vi "Register gRPC Methods.vi"(8 "error in (no error)":errorcluster, 11 "gRPC service in":refnum<class "NI_XNET_CAN_Bus_Monitor_API.lvclass">) -> (0 "error out":errorcluster, 3 "gRPC service out":refnum<class "NI_XNET_CAN_Bus_Monitor_API.lvclass">)   [LabVIEW 2025, in "xnet_can_bus_monitor_api_server.lvlib" / "NI_XNET_CAN_Bus_Monitor_API.lvclass"]
uses:
  NI_XNET_CAN_Bus_Monitor_API.lvclass
  typeDefs/Server Internal UEs.ctl
  typeDefs/Server Internal Message.ctl
  typeDefs/Server gRPC UEs.ctl
  <vilib>/gRPC/LabVIEW gRPC Library/Server API/typeDefs/gRPCId Cluster.ctl
  <vilib>/gRPC/LabVIEW gRPC Library/Shared/grpcId.ctl
  NI_XNET_CAN_Bus_Monitor_API.lvclass/NI_XNET_CAN_Bus_Monitor_API.ctl
  <vilib>/gRPC/LabVIEW gRPC Library/grpc-lvsupport-release.lvlib
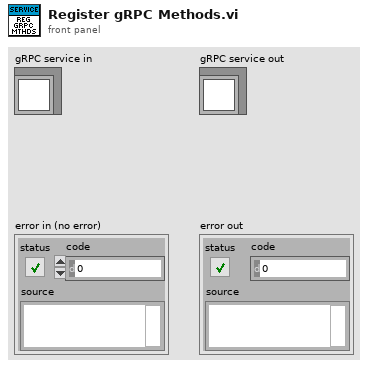
[diagram p1: front panel]
types:
  T1 = typedef "xnet_can_bus_monitor_api_server.lvlib/NI_XNET_CAN_Bus_Monitor_API.lvclass/Server gRPC UEs.ctl" = cluster{"NI_XNET_CAN_Bus_Monitor_API PassThru gRPC UE":refnum<user-event>, "NI_XNET_CAN_Bus_Monitor_API GetStreamingFilter gRPC UE":refnum<user-event>, "NI_XNET_CAN_Bus_Monitor_API SetStreamingFilter gRPC UE":refnum<user-event>, "NI_XNET_CAN_Bus_Monitor_API ResetStreamingFilter gRPC UE":refnum<user-event>, "NI_XNET_CAN_Bus_Monitor_API InitializeSettings gRPC UE":refnum<user-event>, "NI_XNET_CAN_Bus_Monitor_API StopProcess gRPC UE":refnum<user-event>, "NI_XNET_CAN_Bus_Monitor_API StreamBus gRPC UE":refnum<user-event>}
  T2 = typedef "xnet_can_bus_monitor_api_server.lvlib/NI_XNET_CAN_Bus_Monitor_API.lvclass/Server Internal UEs.ctl" = cluster{"NI_XNET_CAN_Bus_Monitor_API PassThru Internal UE":refnum<user-event>, "NI_XNET_CAN_Bus_Monitor_API GetStreamingFilter Internal UE":refnum<user-event>, "NI_XNET_CAN_Bus_Monitor_API SetStreamingFilter Internal UE":refnum<user-event>, "NI_XNET_CAN_Bus_Monitor_API ResetStreamingFilter Internal UE":refnum<user-event>, "NI_XNET_CAN_Bus_Monitor_API InitializeSettings Internal UE":refnum<user-event>, "NI_XNET_CAN_Bus_Monitor_API StopProcess Internal UE":refnum<user-event>, "NI_XNET_CAN_Bus_Monitor_API StreamBus Internal UE":refnum<user-event>}
  T3 = typedef "grpc-lvsupport-release.lvlib/grpcId.ctl" = u64
  T4 = typedef "xnet_can_bus_monitor_api_server.lvlib/NI_XNET_CAN_Bus_Monitor_API.lvclass/Server Internal Message UE.ctl" = refnum<user-event>
  T5 = typedef "grpc-lvsupport-release.lvlib/gRPCId Cluster UE.ctl" = refnum<user-event>
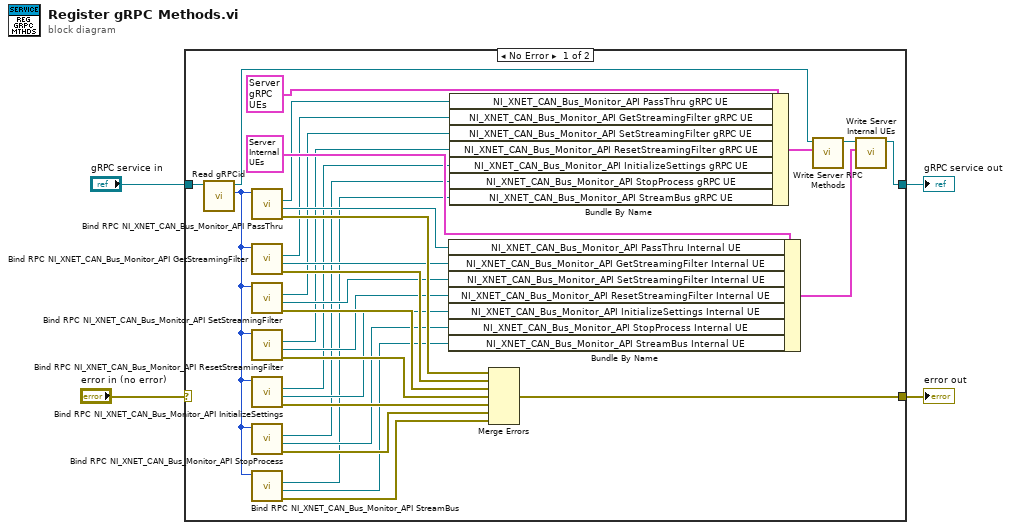
[diagram p0: block diagram]
diagram:
  n1 = case shown="No Error" "error in (no error)" {
    selector: "error in (no error)" -> [_ w36]
    tunnel: "gRPC service in" -> [w27 w37]
    tunnel: [w35 w36] -> w3
    tunnel: [w34 w37] -> w2
    frame No Error {
      n2 = call-dynamic "Read gRPCid.vi"("gRPC service in"=w27) -> ("gRPCid"=w26:T3, "gRPC service out"=w28:refnum<class "NI_XNET_CAN_Bus_Monitor_API.lvclass">)  [unwired: 8 in, 1 out]
      n3 = call "Bind RPC NI_XNET_CAN_Bus_Monitor_API PassThru.vi"("gRPCid server in"=w26) -> ("error out"=w25:errorcluster, "NI_XNET_CAN_Bus_Monitor_API PassThru Internal UE"=w23:T4, "NI_XNET_CAN_Bus_Monitor_API PassThru gRPC UE"=w24:T5)  [unwired: 7 in, 1 out]
      n4 = call "Bind RPC NI_XNET_CAN_Bus_Monitor_API GetStreamingFilter.vi"("gRPCid server in"=w26) -> ("error out"=w22:errorcluster, "NI_XNET_CAN_Bus_Monitor_API GetStreamingFilter Internal UE"=w20:T4, "NI_XNET_CAN_Bus_Monitor_API GetStreamingFilter gRPC UE"=w21:T5)  [unwired: 7 in, 1 out]
      n5 = call "Bind RPC NI_XNET_CAN_Bus_Monitor_API SetStreamingFilter.vi"("gRPCid server in"=w26) -> ("error out"=w19:errorcluster, "NI_XNET_CAN_Bus_Monitor_API SetStreamingFilter Internal UE"=w17:T4, "NI_XNET_CAN_Bus_Monitor_API SetStreamingFilter gRPC UE"=w18:T5)  [unwired: 7 in, 1 out]
      n6 = call "Bind RPC NI_XNET_CAN_Bus_Monitor_API ResetStreamingFilter.vi"("gRPCid server in"=w26) -> ("error out"=w16:errorcluster, "NI_XNET_CAN_Bus_Monitor_API ResetStreamingFilter Internal UE"=w14:T4, "NI_XNET_CAN_Bus_Monitor_API ResetStreamingFilter gRPC UE"=w15:T5)  [unwired: 7 in, 1 out]
      n7 = call "Bind RPC NI_XNET_CAN_Bus_Monitor_API InitializeSettings.vi"("gRPCid server in"=w26) -> ("error out"=w13:errorcluster, "NI_XNET_CAN_Bus_Monitor_API InitializeSettings Internal UE"=w11:T4, "NI_XNET_CAN_Bus_Monitor_API InitializeSettings gRPC UE"=w12:T5)  [unwired: 7 in, 1 out]
      n8 = call "Bind RPC NI_XNET_CAN_Bus_Monitor_API StopProcess.vi"("gRPCid server in"=w26) -> ("error out"=w10:errorcluster, "NI_XNET_CAN_Bus_Monitor_API StopProcess Internal UE"=w8:T4, "NI_XNET_CAN_Bus_Monitor_API StopProcess gRPC UE"=w9:T5)  [unwired: 7 in, 1 out]
      n9 = call "Bind RPC NI_XNET_CAN_Bus_Monitor_API StreamBus.vi"("gRPCid server in"=w26) -> ("error out"=w7:errorcluster, "NI_XNET_CAN_Bus_Monitor_API StreamBus Internal UE"=w5:T4, "NI_XNET_CAN_Bus_Monitor_API StreamBus gRPC UE"=w6:T5)  [unwired: 7 in, 1 out]
      n10 = Bundle By Name ("Bundle Internal UEs")(cluster=T2 {"NI_XNET_CAN_Bus_Monitor_API PassThru Internal UE"=refnum, "NI_XNET_CAN_Bus_Monitor_API GetStreamingFilter Internal UE"=refnum, "NI_XNET_CAN_Bus_Monitor_API SetStreamingFilter Internal UE"=refnum, "NI_XNET_CAN_Bus_Monitor_API ResetStreamingFilter Internal UE"=refnum, "NI_XNET_CAN_Bus_Monitor_API InitializeSettings Internal UE"=refnum, "NI_XNET_CAN_Bus_Monitor_API StopProcess Internal UE"=refnum, "NI_XNET_CAN_Bus_Monitor_API StreamBus Internal UE"=refnum} ("Server Internal UEs"), "NI_XNET_CAN_Bus_Monitor_API PassThru Internal UE"=w23, "NI_XNET_CAN_Bus_Monitor_API GetStreamingFilter Internal UE"=w20, "NI_XNET_CAN_Bus_Monitor_API SetStreamingFilter Internal UE"=w17, "NI_XNET_CAN_Bus_Monitor_API ResetStreamingFilter Internal UE"=w14, "NI_XNET_CAN_Bus_Monitor_API InitializeSettings Internal UE"=w11, "NI_XNET_CAN_Bus_Monitor_API StopProcess Internal UE"=w8, "NI_XNET_CAN_Bus_Monitor_API StreamBus Internal UE"=w5) -> (w33:T2)
      n11 = Bundle By Name ("Bundle gRPC UEs")(cluster=T1 {"NI_XNET_CAN_Bus_Monitor_API PassThru gRPC UE"=refnum, "NI_XNET_CAN_Bus_Monitor_API GetStreamingFilter gRPC UE"=refnum, "NI_XNET_CAN_Bus_Monitor_API SetStreamingFilter gRPC UE"=refnum, "NI_XNET_CAN_Bus_Monitor_API ResetStreamingFilter gRPC UE"=refnum, "NI_XNET_CAN_Bus_Monitor_API InitializeSettings gRPC UE"=refnum, "NI_XNET_CAN_Bus_Monitor_API StopProcess gRPC UE"=refnum, "NI_XNET_CAN_Bus_Monitor_API StreamBus gRPC UE"=refnum} ("gRPC Server Method Events"), "NI_XNET_CAN_Bus_Monitor_API PassThru gRPC UE"=w24, "NI_XNET_CAN_Bus_Monitor_API GetStreamingFilter gRPC UE"=w21, "NI_XNET_CAN_Bus_Monitor_API SetStreamingFilter gRPC UE"=w18, "NI_XNET_CAN_Bus_Monitor_API ResetStreamingFilter gRPC UE"=w15, "NI_XNET_CAN_Bus_Monitor_API InitializeSettings gRPC UE"=w12, "NI_XNET_CAN_Bus_Monitor_API StopProcess gRPC UE"=w9, "NI_XNET_CAN_Bus_Monitor_API StreamBus gRPC UE"=w6) -> (w30:T1)
      n12 = Merge Errors(w25, w22, w19, w16, w13, w10, w7) -> (w35:errorcluster)
      n13 = call "Write Server RPC Methods.vi"("Server RPC Methods"=w30, "gRPC service in"=w28) -> ("gRPC service out"=w31:refnum<class "NI_XNET_CAN_Bus_Monitor_API.lvclass">)  [unwired: 8 in, 1 out]
      n14 = call "Write Server Internal UEs.vi"("Server Internal UEs"=w33, "gRPC service in"=w31) -> ("gRPC service out"=w34:refnum<class "NI_XNET_CAN_Bus_Monitor_API.lvclass">)  [unwired: 8 in, 1 out]
    }
    frame Error {
    }
  }
  "error out" <- w3
  "gRPC service out" <- w2
